vi "Close.vi"(8 "error in":errorcluster, 11 "DB-ADO in":refnum<class "DB-ADO.lvclass">) -> (0 "error out":errorcluster, 3 "DB-ADO out":refnum<class "DB-ADO.lvclass">)   [LabVIEW 2020, in "hse-db-ado.lvlib" / "DB-ADO.lvclass"]
doc: "Close the ADO connection.\n\n____\nHAMPEL SOFTWARE ENGINEERING v1.4.0 (2023-12-19 09:52)"
uses:
  DB-ADO.lvclass
  DB-ADO.lvclass/DB-ADO.ctl
  ADO-DB-Drivers/ADO-DB-Driver.lvlib
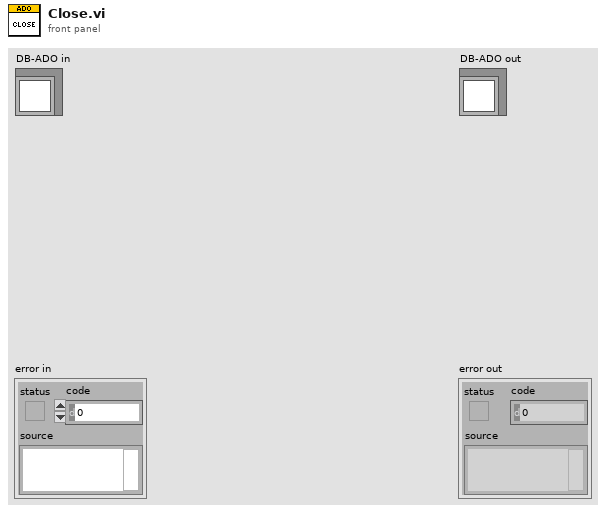
[diagram p1: front panel]
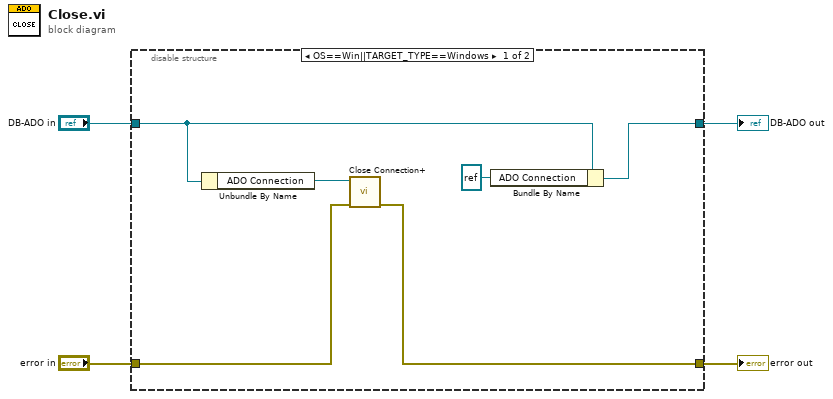
[diagram p0: block diagram]
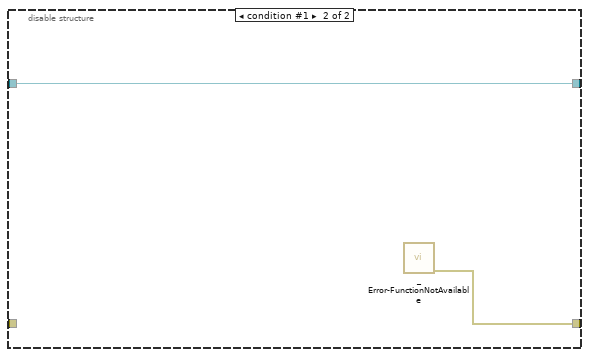
[diagram p2: hidden frame]
diagram:
  n1 = disable-structure shown="OS==Win||TARGET_TYPE==Windows" {
    disable-tunnel: "error in" -> [w9 _]
    disable-tunnel: [w8 w11] -> w3
    disable-tunnel: "DB-ADO in" -> [w7 w12]
    disable-tunnel: [w6 w12] -> w1
    frame condition #0 (active) {
      n2 = Unbundle By Name(w7) -> ("ADO Connection"=w10:refnum<k7>)
      n3 = call "Close Connection+.vi"("error in"=w9, "Connection"=w10) -> ("error out"=w8:errorcluster)  [unwired: 5 in]
      n4 = Bundle By Name(cluster=w7, "ADO Connection"=refnum<k7> refnum) -> (w6:refnum<class "DB-ADO.lvclass">)
    }
    frame condition #1 {
      n5 = call "_Error-FunctionNotAvailable.vi"() -> ("error out"=w11:errorcluster)  [unwired: 11 in]
    }
  }
  "error out" <- w3
  "DB-ADO out" <- w1
